vi "write meta file.vi"(8 "error in":errorcluster, 9 "metadata":T1[](array[typedef]), 10 "file basename":string, 11 "output folder":path) -> (0 "error out":errorcluster)   [LabVIEW 2020]
uses:
  metadata.ctl
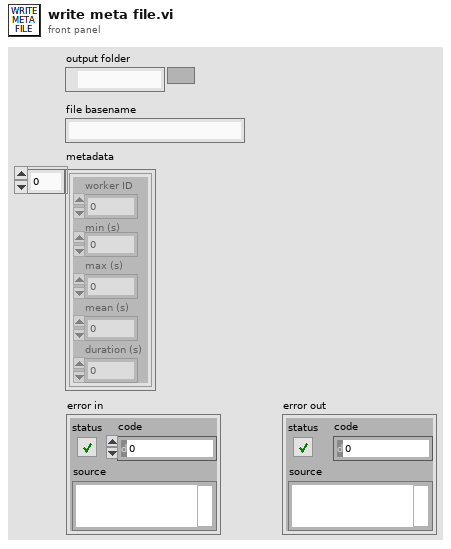
[diagram p1: front panel]
types:
  T1 = typedef "metadata.ctl" = cluster{"worker ID":u32, "min (s)":dbl, "max (s)":dbl, "mean (s)":dbl, "duration (s)":dbl}
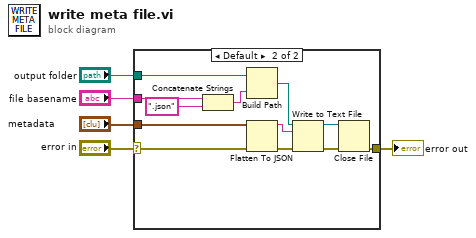
[diagram p0: block diagram]
diagram:
  n1 = case shown="Default" "error in" {
    selector: "error in" -> [_ w8]
    tunnel: [_ w12] -> w5
    tunnel: "file basename" -> [_ w10]
    tunnel: "output folder" -> [_ w9]
    tunnel: "metadata" -> [_ w6]
    frame No Error {
    }
    frame Default {
      n2 = Concatenate Strings(w10, ".json" ("string")) -> (w11:string)
      n3 = Build Path(base path=w9, name or relative path=w11) -> (appended path=w15:path)
      n4 = Flatten To JSON(anything=w6, error in (no error)=w8) -> (JSON string=w16:string, 11:w17:errorcluster)  [unwired: 1 in]
      n5 = Write to Text File(file (use dialog)=w15, text=w16, error in=w17) -> (refnum out=w13:refnum<file>, error out=w14:errorcluster)  [unwired: 1 in, 1 out]
      n6 = Close File(refnum=w13, error in=w14) -> (error out=w12:errorcluster)  [unwired: 1 out]
    }
  }
  "error out" <- w5
